vi "Robot_Simulation_Connect_Listen.vi"(8 "error in (no error)":errorcluster, 10 "timeout ms (25000)":i32, 11 "port":u16) -> (0 "error out":errorcluster, 1 "Properties:Request URI":string, 2 "Properties:Return Headers":variant, 3 "WebSocket Connection out":refnum<class "websocket server.lvclass">)   [LabVIEW 2020]
uses:
  <vilib>/mediamongrels ltd/websockets/websockets/websocket server/websocket server.lvclass
  C:/Program Files (x86)/National Instruments/LabVIEW 2020/vi.lib/mediamongrels ltd/websockets/websockets/websocket/websocket.lvclass
  <vilib>/mediamongrels ltd/websockets/websockets/websocket/websocket.lvclass/websocket.ctl
  <vilib>/mediamongrels ltd/websockets/websockets/websocket server/websocket server.lvclass/websocket server.ctl
  <vilib>/mediamongrels ltd/websockets/websockets/websocket/read return headers.vi
  <vilib>/mediamongrels ltd/websockets/websockets/websocket server/read request uri.vi
  <vilib>/mediamongrels ltd/websockets/sockets/visa tcp listener/visa tcp listener.lvclass
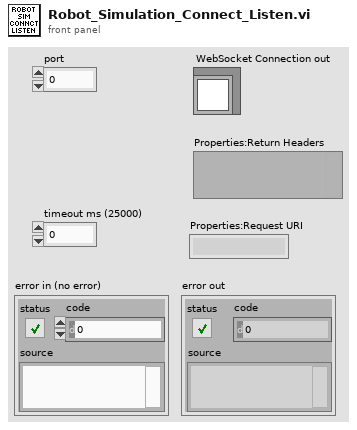
[diagram p1: front panel]
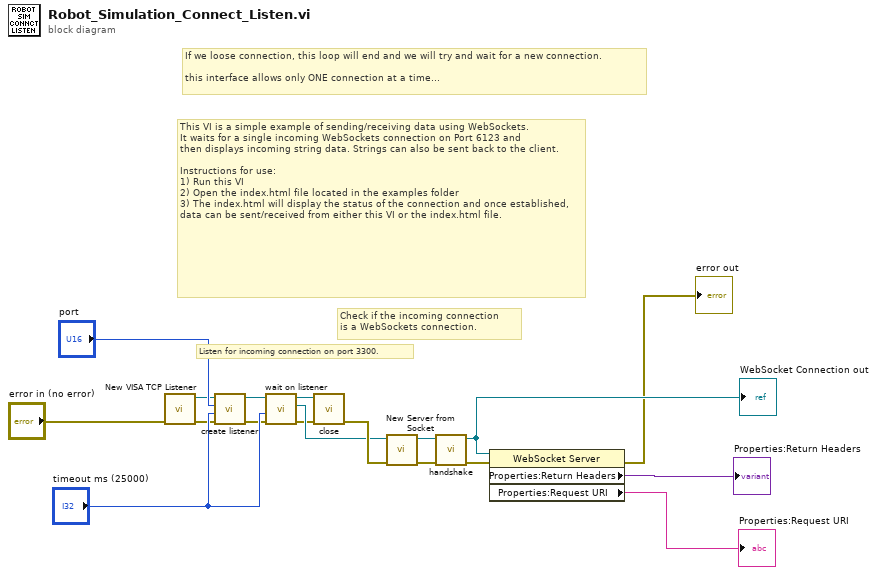
[diagram p0: block diagram]
diagram:
  # "If we loose connection, this loop will end and we will try and wait for a new connection.\n\nthis interface allows only ONE connection at a time..."
  # "This VI is a simple example of sending/receiving data using WebSockets.\nIt waits for a single incoming WebSockets connection on Port 6123 and\nthen displays incoming string data. Strings can also be sent back to the client.\n\nInstructions for use:\n1) Run this VI\n2) Open the index.html file located in the examples folder\n3) The index.html will display the status of the connection and once established, data can be sent/received from either this VI or the index.html file."
  # "Check if the incoming connection\nis a WebSockets connection."
  # "Listen for incoming connection on port 3300."
  n1 = call <vilib>:"New VISA TCP Listener.vi"("error in (no error)"="error in (no error)") -> ("error out"=w9:errorcluster, "VISA TCP Listener out"=w8:refnum<class "visa tcp listener.lvclass">)  [unwired: 9 in]
  n2 = call-dynamic "create listener.vi"("error in (no error)"=w9, "timeout ms (5000)"="timeout ms (25000)", "Port"="port", "VISA TCP Listener in"=w8) -> ("error out"=w11:errorcluster, "VISA TCP Listener out"=w13:refnum<class "visa tcp listener.lvclass">)  [unwired: 6 in]
  n3 = call-dynamic "wait on listener.vi"("error in (no error)"=w11, "timeout ms (5000)"="timeout ms (25000)", "VISA TCP Listener in"=w13) -> ("error out"=w10:errorcluster, "Socket out"=w16:refnum<class "socket.lvclass">, "VISA TCP Listener out"=w12:refnum<class "visa tcp listener.lvclass">)  [unwired: 6 in]
  n4 = call-dynamic "close.vi"("error in (no error)"=w10, "VISA TCP Listener in"=w12) -> ("error out"=w17:errorcluster)  [unwired: 9 in]
  n5 = call <vilib>:"New Server from Socket.vi"("error in (no error)"=w17, "Socket"=w16) -> ("error out"=w5:errorcluster, "WebSocket Server out"=w4:refnum<class "websocket server.lvclass">)  [unwired: 8 in]
  n6 = call-dynamic "handshake.vi"("error in (no error)"=w5, "WebSocket Connection in"=w4) -> ("error out"=w3:errorcluster, "WebSocket Connection out"=w18:refnum<class "websocket server.lvclass">)  [unwired: 8 in]
  "WebSocket Connection out" <- w18
  n7 = property class="WebSocket Server"(reference=w18, error in=w3) -> (error out=→"error out":errorcluster, "Properties:Return Headers"=→"Properties:Return Headers":variant, "Properties:Request URI"=→"Properties:Request URI":string)  [unwired: 1 out]
